vi "control loop process action.vi"(11 "control loop data in":T1) -> (3 "control loop data out":T1)   [LabVIEW 2013, in "main engine.lvlib"]
doc: "This VI calls the input method of any modules specified using the 'Input Method Indices' if the 'Execute?' flag for the method is TRUE. It also exchanges the data necessary for that method with the data in the main engine tags. Any errors that occur are stored to be handled at the end of the engine's execution."
uses:
  main engine.lvlib
  control loop data.ctl
  <vilib>/NI/Tag Bus/table/data table.ctl
  engine run schedule.ctl
  engine decimation schedule.ctl
  full module data.ctl
  <vilib>/NI/Tag Bus Module Framework/runtime/TBM module execution interface.lvclass
  module run state.ctl
  async executor/asynchronous executor reference.ctl
  async executor/async message to executor.ctl
  Runtime/async command notification.ctl
  Runtime/async error info.ctl
  <vilib>/NI/Tag Bus Module Framework/runtime/error classification.ctl
  <vilib>/NI/Tag Bus Module Framework/module configuration/TBM module configuration.lvclass
  module method data.ctl
  <vilib>/NI/Tag Bus/table/transfer specification.ctl
  <vilib>/NI/Tag Bus/tag/Data Type.ctl
  fault handling spec.ctl
  Configuration/Error Actions.ctl
  <vilib>/NI/Tag Bus/table/data table.lvlib
  <vilib>/NI/Tag Bus/tag/tag descriptor.lvclass
  Configuration/Standard Engine Configuration.lvclass
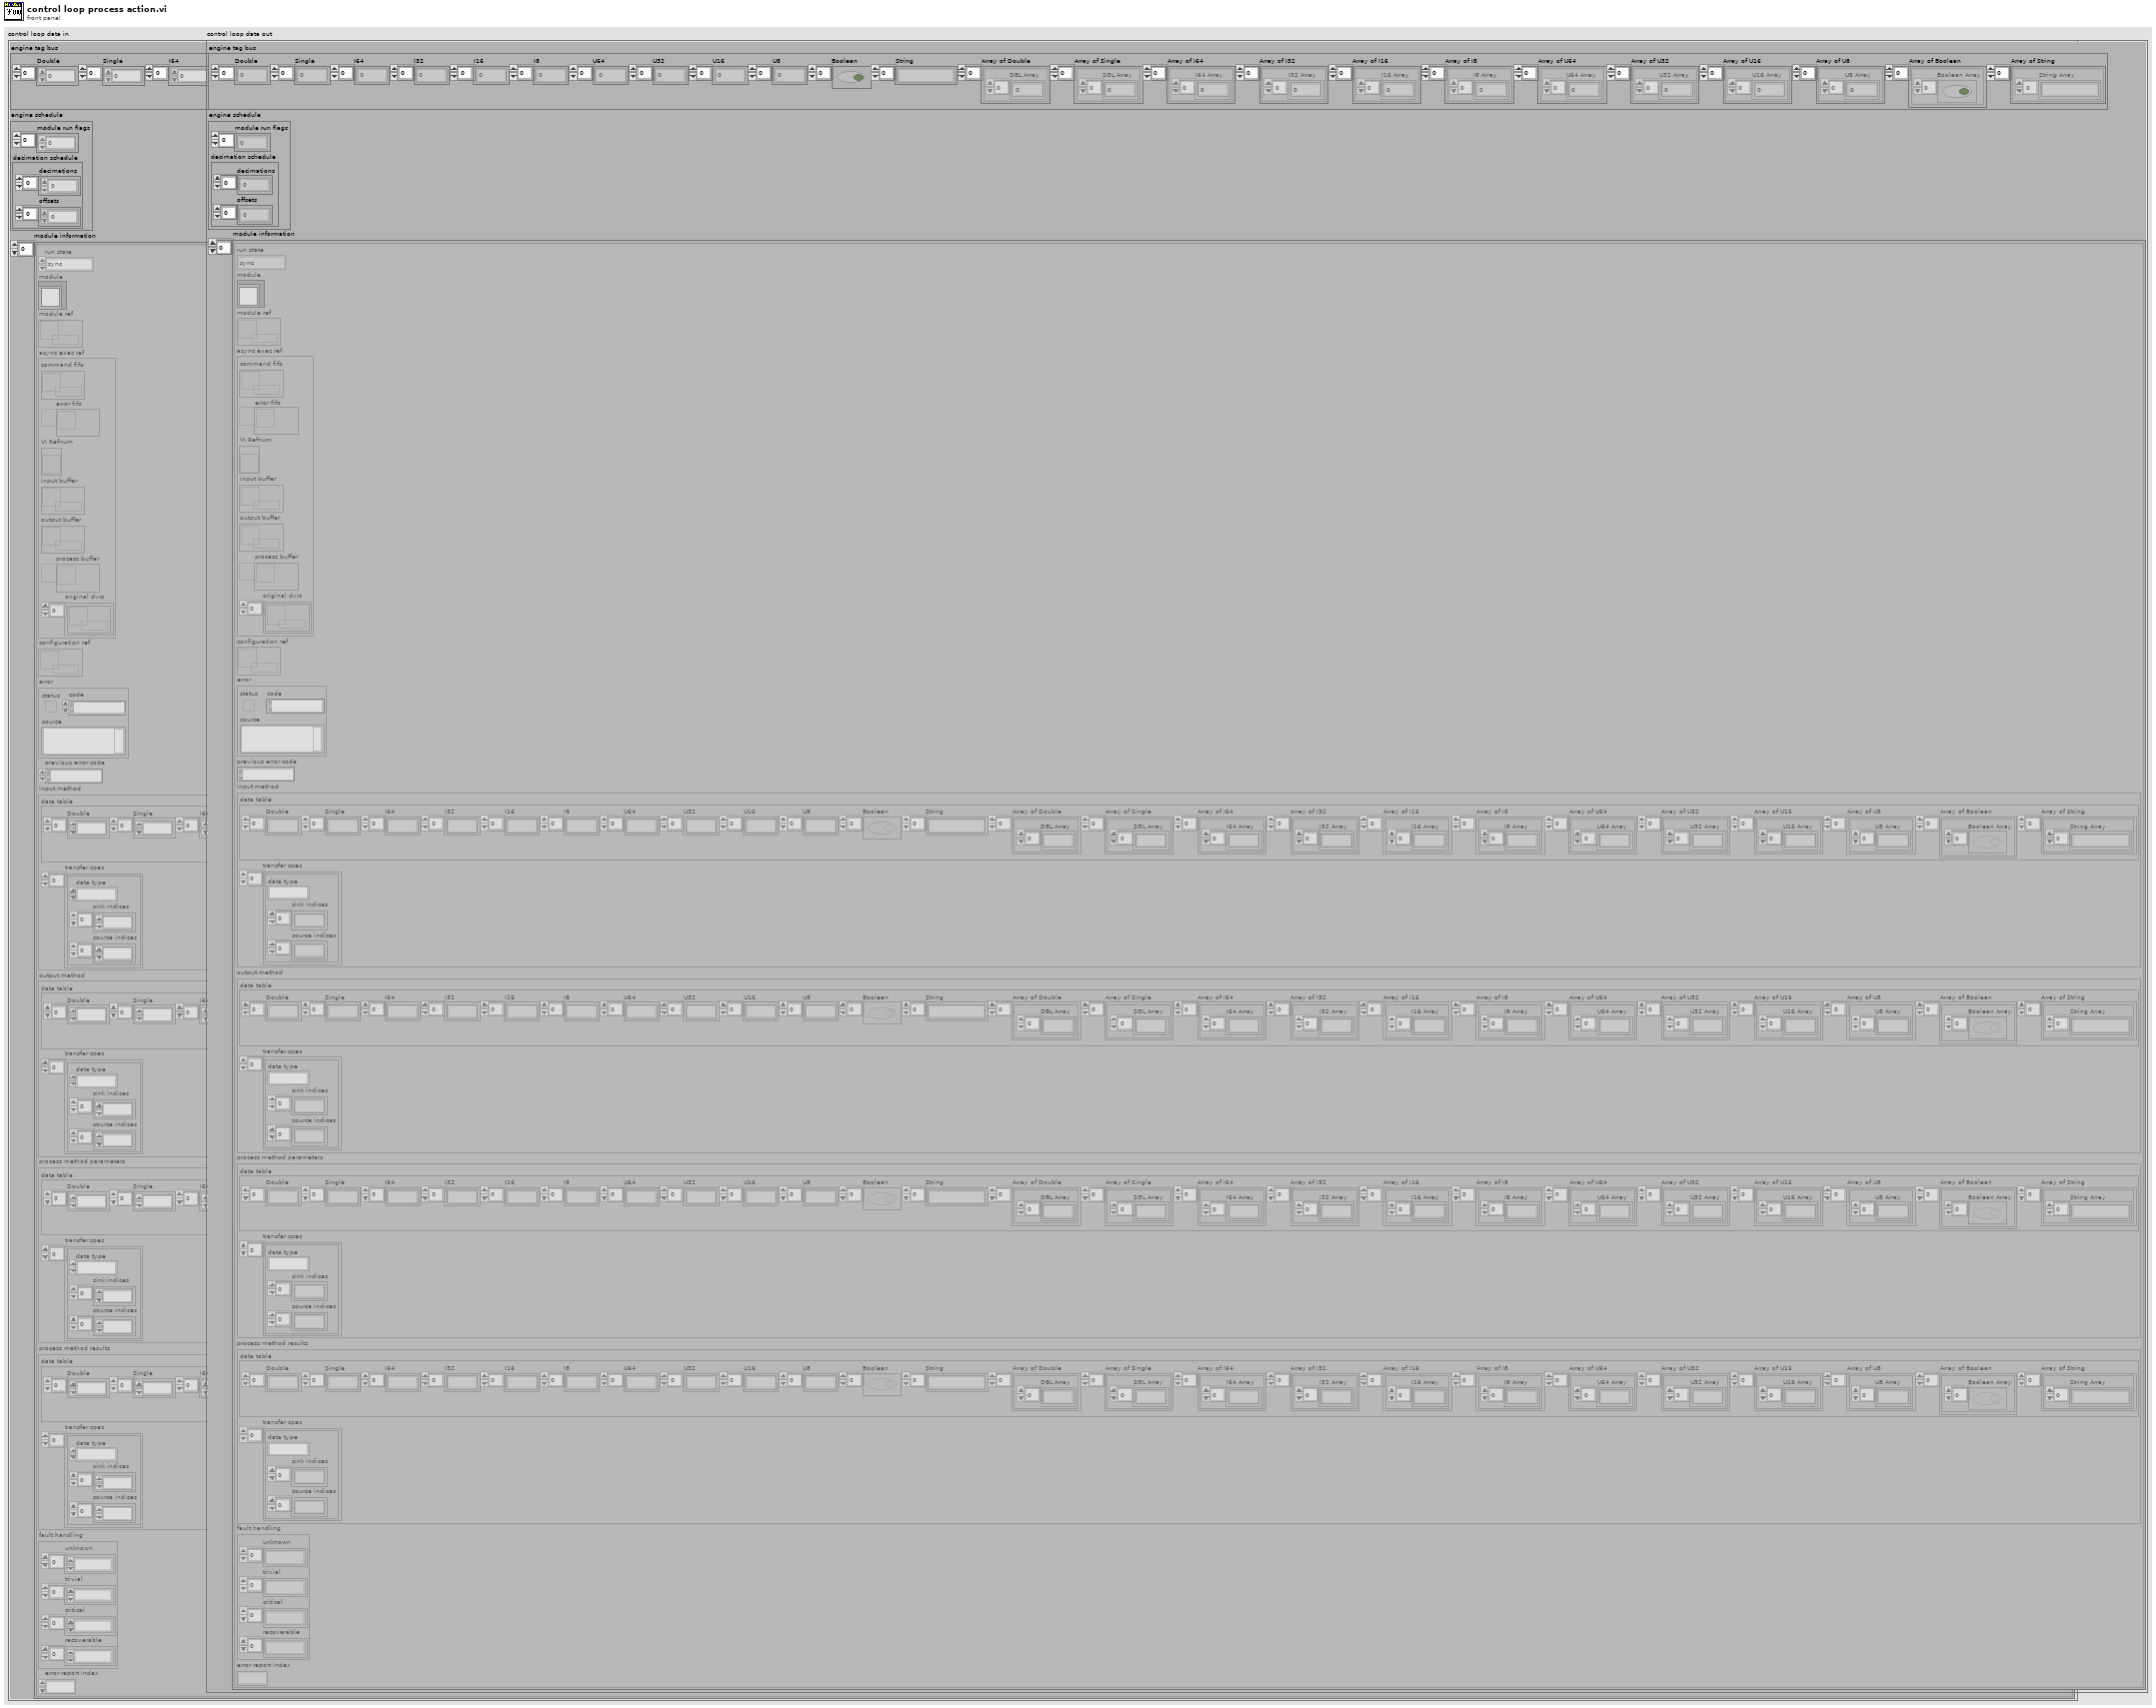
[diagram p1: front panel]
types:
  T1 = typedef "main engine.lvlib/control loop data.ctl" = cluster{"engine tag bus":T2, "engine schedule":T3, "module information":T5[]}
  T2 = typedef "tag bus.lvlib/data table.lvlib/data table.ctl" = cluster{"Double":dbl[], "Single":sgl[], "I64":i64[], "I32":i32[], "I16":i16[], "I8":i8[], "U64":u64[], "U32":u32[], "U16":u16[], "U8":u8[], "Boolean":bool[], "String":string[], "Array of Double":cluster{"DBL Array":dbl[]}[], "Array of Single":cluster{"SGL Array":sgl[]}[], "Array of I64":cluster{"I64 Array":i64[]}[], "Array of I32":cluster{"I32 Array":i32[]}[], "Array of I16":cluster{"I16 Array":i16[]}[], "Array of I8":cluster{"I8 Array":i8[]}[], "Array of U64":cluster{"U64 Array":u64[]}[], "Array of U32":cluster{"U32 Array":u32[]}[], "Array of U16":cluster{"U16 Array":u16[]}[], "Array of U8":cluster{"U8 Array":u8[]}[], "Array of Boolean":cluster{"Boolean Array":bool[]}[], "Array of String":cluster{"String Array":string[]}[]}
  T3 = typedef "main engine.lvlib/engine run schedule.ctl" = cluster{"module run flags":u8[], "decimation schedule":T4}
  T4 = typedef "main engine.lvlib/engine decimation schedule.ctl" = cluster{"decimations":u16[], "offsets":u16[]}
  T5 = typedef "main engine.lvlib/full module data.ctl" = cluster{"run state":T6, "module":refnum<class "TBM module execution interface.lvclass">, "module ref":refnum<data-value>, "async exec ref":T7, "configuration ref":refnum<data-value>, "error":errorcluster, "previous error code":i32, "input method":T8, "output method":T8, "process method parameters":T8, "process method results":T8, "fault handling":T11, "error report index ":i32}
  T6 = typedef "main engine.lvlib/module run state.ctl" = enum16{"sync", "async"}
  T7 = typedef "main engine.lvlib/asynchronous executor reference.ctl" = cluster{"command fifo":refnum<k33>, "error fifo":refnum<k33>, "VI Refnum":refnum<vi>, "input buffer":refnum<k33>, "output buffer":refnum<k33>, "process buffer":refnum<k33>, "original dvrs":refnum<data-value>[]}
  T8 = typedef "main engine.lvlib/module method data.ctl" = cluster{"data table":T2, "transfer spec":T9[]}
  T9 = typedef "tag bus.lvlib/data table.lvlib/transfer specification.ctl" = cluster{"data type":T10, "sink indices":i32[], "source indices":i32[]}
  T10 = typedef "tag bus.lvlib/tag descriptor.lvclass/Data Type.ctl" = enum16{"Double", "Single", "I64", "I32", "I16", "I8", "U64", "U32", "U16", "U8", "Boolean", "String", "Array of Double", "Array of Single", "Array of I64", "Array of I32", "Array of I16", "Array of I8", "Array of U64", "Array of U32", "Array of U16", "Array of U8", "Array of Boolean", "Array of String"}
  T11 = typedef "main engine.lvlib/fault handling spec.ctl" = cluster{"unknown":T12[], "trivial":T12[], "critical":T12[], "recoverable":T12[]}
  T12 = typedef "Standard Engine Configuration.lvclass/Error Actions.ctl" = enum16{"Clear", "Notify", "Stop Component", "Stop Engine", "Safe State", "Attempt Recovery"}
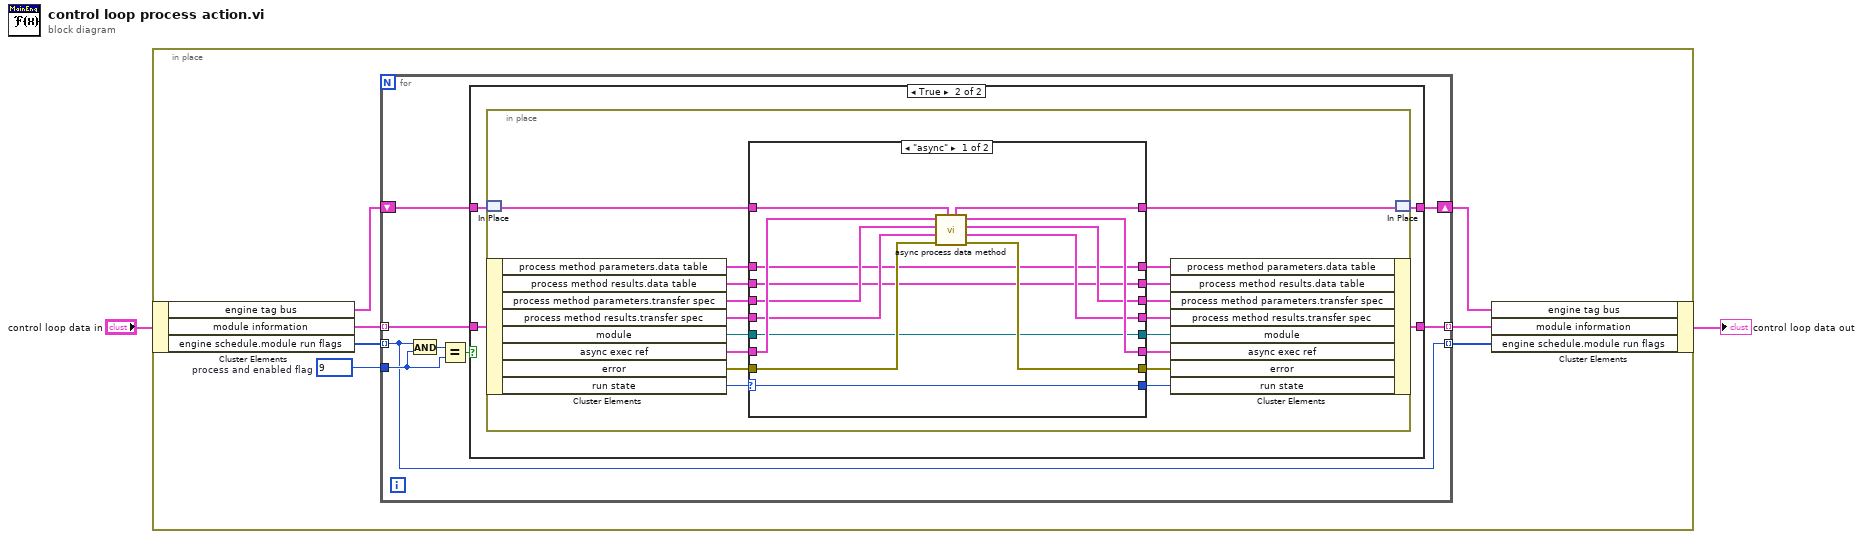
[diagram p0: block diagram]
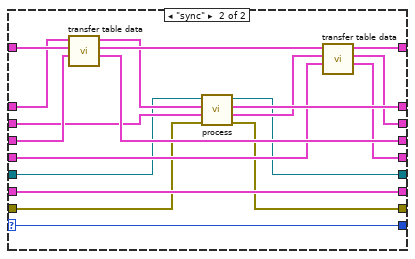
[diagram p3: hidden frame]
diagram:
  n1 = in-place {
    w4 = u8 9  # process and enabled flag
    n2 = in-place-cluster #1("control loop data in") -> ("engine tag bus"=w8:T2, "module information"=w6:T5[], "engine schedule.module run flags"=w9:u8[])
    n3 = for {
      tunnel: w9 -> [w10] mode=indexing
      shift-right: [w16] -> w7
      shift-left: w8 -> [w17]
      tunnel: w6 -> [w15] mode=indexing
      tunnel: [w14] -> w5 mode=indexing
      tunnel: w4 -> [w12]
      tunnel: [w10] -> w3 mode=indexing
      n4 = And(x=w10, y=w12) -> (x .and. y?=w13:u8)
      n5 = Equal?(x=w13, y=w12) -> (x = y?=w11:bool)
      n6 = case shown="True" w11 {
        tunnel: w17 -> [w19 w23]
        tunnel: [w19 w22] -> w16
        tunnel: w15 -> [w18 w21]
        tunnel: [w18 w20] -> w14
        frame False {
        }
        frame True {
          n7 = in-place {
            n8 = in-place-match #2(w23) -> (w39:T2)
            n9 = in-place-cluster #3(w21) -> ("process method parameters.data table"=w27:T2, "process method results.data table"=w26:T2, "process method parameters.transfer spec"=w28:T9[], "process method results.transfer spec"=w38:T9[], "module"=w37:refnum<class "TBM module execution interface.lvclass">, "async exec ref"=w34:T7, "error"=w33:errorcluster, "run state"=w41:T6)
            n10 = case shown="\"async\"" w41 {
              selector: w41 -> [w55 w74]
              tunnel: [w53 w70] -> w40
              tunnel: w39 -> [w54 w72]
              tunnel: w38 -> [w45 w64]
              tunnel: w37 -> [w48 w59]
              tunnel: [w48 w56] -> w36
              tunnel: [w49 w73] -> w35
              tunnel: w34 -> [w52 w73]
              tunnel: w33 -> [w51 w58]
              tunnel: [w50 w57] -> w32
              tunnel: [w55 w74] -> w31
              tunnel: [w47 w67] -> w30
              tunnel: [w46 w61] -> w29
              tunnel: w28 -> [w44 w68]
              tunnel: w27 -> [w43 w69]
              tunnel: w26 -> [w42 w60]
              tunnel: [w43 w65] -> w25
              tunnel: [w42 w62] -> w24
              frame "async" {
                n11 = call "async process data method.vi"("engine tag data in"=w54, "error in"=w51, "result transfers in"=w45, "parameter transfers in"=w44, "async exec in"=w52) -> ("error out"=w50:errorcluster, "result transfers out"=w46:T9[], "parameter transfers out"=w47:T9[], "async exec out"=w49:T7, "engine tag data out"=w53:T2)  [unwired: 2 in]
              }
              frame "sync" {
                n12 = call <vilib>:"transfer table data.vi"("transfer specification in"=w68, "data table source in"=w72, "data table sink in"=w69) -> ("transfer specification out"=w67:T9[], "data table source out"=w71:T2, "data table sink out"=w66:T2)  [unwired: 6 in]
                n13 = call-dynamic "process.vi"("error in"=w58, "result allocation"=w60, "parameters"=w66, "module in"=w59) -> ("error out"=w57:errorcluster, "results"=w63:T2, "parameter allocation"=w65:T2, "module out"=w56:refnum<class "TBM module execution interface.lvclass">)  [unwired: 4 in]
                n14 = call <vilib>:"transfer table data.vi"("transfer specification in"=w64, "data table source in"=w63, "data table sink in"=w71) -> ("transfer specification out"=w61:T9[], "data table source out"=w62:T2, "data table sink out"=w70:T2)  [unwired: 6 in]
              }
            }
            n15 = in-place-cluster #3("process method parameters.data table"=w25, "process method results.data table"=w24, "process method parameters.transfer spec"=w30, "process method results.transfer spec"=w29, "module"=w36, "async exec ref"=w35, "error"=w32, "run state"=w31) -> (w20:T5)
            n16 = in-place-match #2(w40) -> (w22:T2)
          }
        }
      }
    }
    n17 = in-place-cluster #1("engine tag bus"=w7, "module information"=w5, "engine schedule.module run flags"=w3) -> (→"control loop data out":T1)
  }
